vi "Draw.vi"(0 "FSM.EdgeEnd":refnum<class "FSM.EdgeEnd.lvclass">, 7 "picture in":picture, 9 "location":cluster{"x":i16, "y":i16}, 11 "direction":cluster{"x":i16, "y":i16}) -> (8 "picture out":picture)   [LabVIEW 2020, in "FSM.EdgeEnd.lvclass"]
uses:
  FSM.EdgeEnd.lvclass
  FSM.EdgeEnd.lvclass/FSM.EdgeEnd.ctl
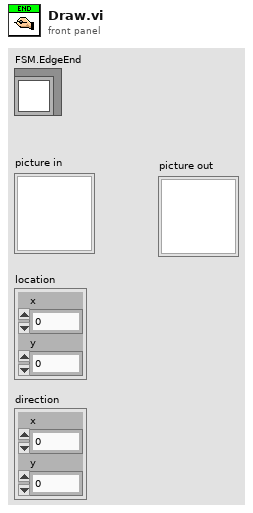
[diagram p1: front panel]
types:
  T1 = cluster{"Width":u16, "Style":enum32{"Solid", "Dash", "Dot", "DashDot", "DashDotDot"}}
  T2 = typedef "FSM.EdgeEnd.lvclass/EndStyle.ctl" = enum16{"Plain", "Arrow", "Box", "Circle", "Diamond"}
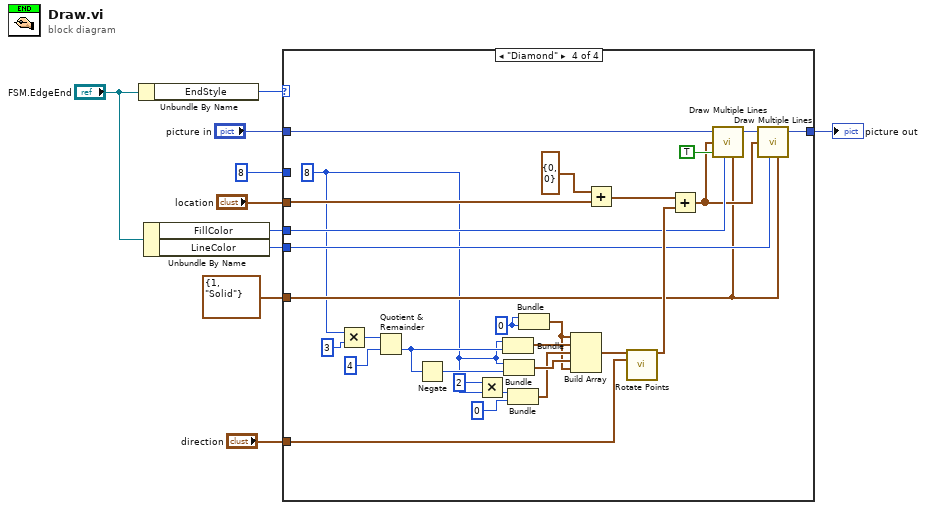
[diagram p0: block diagram]
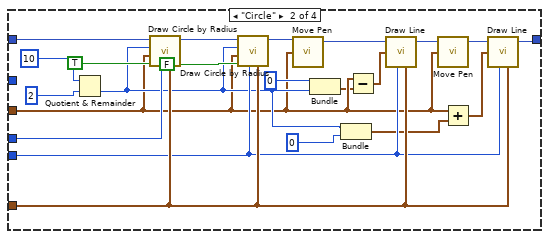
[diagram p3: hidden frame]
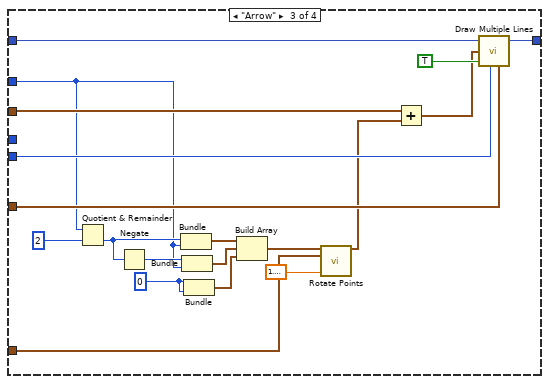
[diagram p4: hidden frame]
diagram:
  n1 = Unbundle By Name("FSM.EdgeEnd") -> ("EndStyle"=w10:T2)
  n2 = Unbundle By Name("FSM.EdgeEnd") -> ("FillColor"=w6:u32, "LineColor"=w5:u32)
  n3 = case shown="\"Diamond\"" w10 {
    tunnel: "location" -> [_ w13 w43 w77]
    tunnel: T1 {"Width"=1, "Style"=enum."Solid"} ("pen") -> [_ w19 w50 w68]
    tunnel: "picture in" -> [w11 w33 w52 w80]
    tunnel: w6 -> [_ w32 _ w73]
    tunnel: w5 -> [_ w18 w48 w69]
    tunnel: [w11 w20 w51 w71] -> w4
    tunnel: 8 -> [_ _ w38 _]
    tunnel: "direction" -> [_ _ w36 w75]
    frame "Plain", Default {
    }
    frame "Circle" {
      n4 = Quotient & Remainder(x=10, y=2) -> (floor(x/y)=w14:i32)  [unwired: 1 out]
      n5 = call <vilib>:"Draw Circle by Radius.vi"("pen"=w19, "color(black)"=w32, "fill?(F)"=TRUE, "pixel center"=w13, "radius"=w14, "picture"=w33) -> ("new picture"=w30:picture)  [unwired: 5 in]
      n6 = call <vilib>:"Draw Circle by Radius.vi"("pen"=w19, "color(black)"=w18, "fill?(F)"=FALSE, "pixel center"=w13, "radius"=w14, "picture"=w30) -> ("new picture"=w26:picture)  [unwired: 5 in]
      n7 = call <vilib>:"Move Pen.vi"("new position"=w13, "picture"=w26) -> ("new picture"=w25:picture)  [unwired: 3 in]
      n8 = Bundle(0, w14) -> (w12:cluster{i32, i32})  [unwired: 1 in]
      n9 = Bundle(w14, 0) -> (w15:cluster{i32, i32})  [unwired: 1 in]
      n10 = Subtract(x=w13, y=w12) -> (x-y=w23:cluster{i32, i32})
      n11 = call <vilib>:"Draw Line.vi"("picture"=w25, "end point"=w23, "color(black)"=w18, "pen"=w19) -> ("new picture"=w22:picture)  [unwired: 5 in]
      n12 = call <vilib>:"Move Pen.vi"("new position"=w13, "picture"=w22) -> ("new picture"=w21:picture)  [unwired: 3 in]
      n13 = Add(x=w13, y=w15) -> (x+y=w17:cluster{i32, i32})
      n14 = call <vilib>:"Draw Line.vi"("picture"=w21, "end point"=w17, "color(black)"=w18, "pen"=w19) -> ("new picture"=w20:picture)  [unwired: 5 in]
    }
    frame "Arrow" {
      w41 = 0
      n15 = Quotient & Remainder(x=w38, y=2) -> (floor(x/y)=w39:i32)  [unwired: 1 out]
      n16 = Negate(x=w39) -> (-x=w40:i32)
      n17 = Bundle(w39, w38) -> (w46:cluster{i32, i32})  [unwired: 1 in]
      n18 = Bundle(w40, w38) -> (w45:cluster{i32, i32})  [unwired: 1 in]
      n19 = Bundle(w41, w41) -> (w44:cluster{i32, i32})  [unwired: 1 in]
      n20 = Build Array(w46, w45, w44) -> (w37:cluster{i32, i32}[])
      n21 = call "Rotate Points.vi"("Points In"=w37, "direction"=w36, "angle"=1.5707963267948966) -> ("Rotated Points"=w35:cluster{i32, i32}[])  [unwired: 12 in]
      n22 = Add(x=w43, y=w35) -> (x+y=w42:cluster{i32, i32}[])
      n23 = call <vilib>:"Draw Multiple Lines.vi"("picture"=w52, "line endpoints"=w42, "fill?(F)"=TRUE, "color(black)"=w48, "pen"=w50) -> ("new picture"=w51:picture)  [unwired: 4 in]
    }
    frame "Diamond" {
      w55 = 8
      w56 = 0
      n24 = Multiply(x=w55, y=3) -> (x*y=w62:i32)
      n25 = Quotient & Remainder(x=w62, y=4) -> (floor(x/y)=w64:i32)  [unwired: 1 out]
      n26 = Negate(x=w64) -> (-x=w65:i32)
      n27 = Multiply(x=2, y=w55) -> (x*y=w54:i32)
      n28 = Bundle(w55, w64) -> (w78:cluster{i32, i32})  [unwired: 1 in]
      n29 = Bundle(w55, w65) -> (w67:cluster{i32, i32})  [unwired: 1 in]
      n30 = Bundle(w54, 0) -> (w66:cluster{i32, i32})  [unwired: 1 in]
      n31 = Bundle(w56, w56) -> (w63:cluster{i32, i32})  [unwired: 1 in]
      n32 = Build Array(w63, w78, w66, w67, w63) -> (w76:cluster{i32, i32}[])
      n33 = Add(x=cluster{"x":i16, "y":i16} {"x"=0, "y"=0}, y=w77) -> (x+y=w58:cluster{"x":i16, "y":i16})
      n34 = call "Rotate Points.vi"("Points In"=w76, "direction"=w75) -> ("Rotated Points"=w74:cluster{i32, i32}[])  [unwired: 13 in]
      n35 = Add(x=w58, y=w74) -> (x+y=w70:cluster{i32, i32}[])
      n36 = call <vilib>:"Draw Multiple Lines.vi"("picture"=w80, "line endpoints"=w70, "fill?(F)"=TRUE, "color(black)"=w73, "pen"=w68) -> ("new picture"=w72:picture)  [unwired: 4 in]
      n37 = call <vilib>:"Draw Multiple Lines.vi"("picture"=w72, "line endpoints"=w70, "color(black)"=w69, "pen"=w68) -> ("new picture"=w71:picture)  [unwired: 5 in]
    }
  }
  "picture out" <- w4
